vi "{{Msg}}Wrapper.vi"(6 "Error":errorcluster, 7 "Layer":T10, 9 "Payload":T9, 10 "MsgAttribs":T6 {"AbsoluteTime" format="%<%x %.3X>T"}, 11 "Actor":T1) -> (1 "Payload":T9, 2 "MsgAttribs":T6 {"AbsoluteTime" format="%<%x %.3X>T"}, 3 "Actor":T1, 4 "Error":errorcluster, 5 "Layer":T10)   [LabVIEW 2020, in "_Template.lvlib" / "{{Msg}}.lvlib"]
uses:
  {{Msg}}.lvlib
  ActorMsg/ActorMsg.lvclass
  jettl/jettl/Actor/Actor.lvclass
  jettl/jettl/Origin.ctl
  jettl/jettl/jettl.lvlib
  jettl/jettl/Lifecycle.ctl
  jettl/jettl/Metadata/Metadata.lvclass
  jettl/jettl/MsgAttribs.ctl
  jettl/jettl/Msg/Msg.lvclass
  jettl/jettl/Msg.ctl
  jettl/jettl/PostSetup.ctl
  jettl/jettl/PreSetup.ctl
  jettl/jettl/MsgNames.ctl
  jettl/jettl/ActorAttribs.ctl
  jettl/jettl/ChildActors.ctl
  jettl/jettl/Actor.ctl
  Payload.ctl
  jettl/jettl/Layer.ctl
  jettl/jettl/MsgExecuteType.ctl
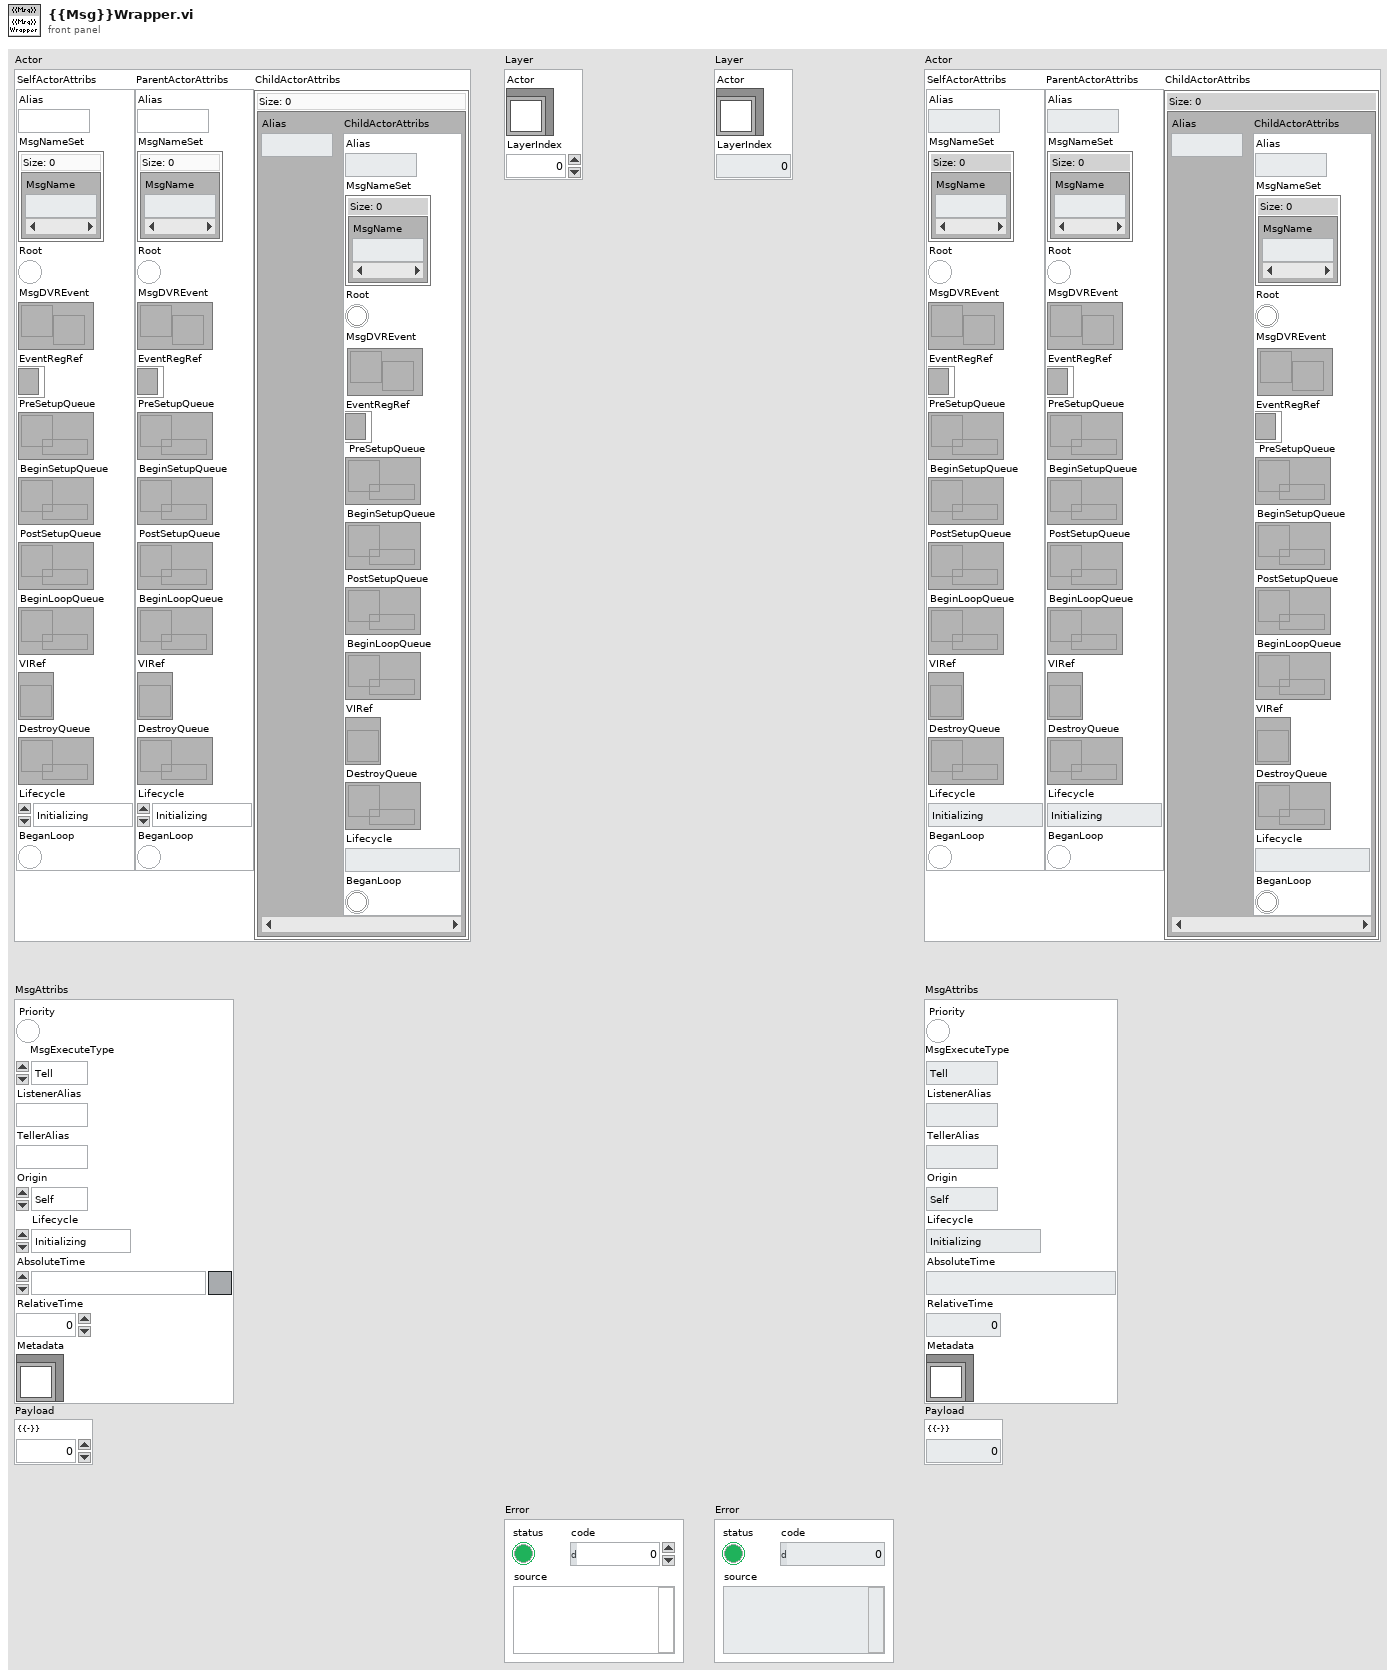
[diagram p1: front panel]
types:
  T1 = typedef "jettl.lvlib/Actor.ctl" = cluster{"SelfActorAttribs":T2, "ParentActorAttribs":T2, "ChildActorAttribs":T5}
  T2 = typedef "jettl.lvlib/ActorAttribs.ctl" = cluster{"Alias":string, "MsgNameSet":T3, "Root":bool, "MsgDVREvent":refnum<user-event>, "EventRegRef":refnum<event-registration>, "PreSetupQueue":refnum<queue>, "BeginSetupQueue":refnum<queue>, "PostSetupQueue":refnum<queue>, "BeginLoopQueue":refnum<queue>, "VIRef":refnum<vi>, "DestroyQueue":refnum<queue>, "Lifecycle":T4, "BeganLoop":bool}
  T3 = typedef "jettl.lvlib/MsgNames.ctl" = set{string}
  T4 = typedef "jettl.lvlib/Lifecycle.ctl" = enum16{"Initializing", "SettingUp", "Starting", "Running", "Stopping", "TearingDown", "Terminated"}
  T5 = typedef "jettl.lvlib/ChildActors.ctl" = map{string, T2}
  T6 = typedef "jettl.lvlib/MsgAttribs.ctl" = cluster{"Priority":bool, "MsgExecuteType":T7, "ListenerAlias":string, "TellerAlias":string, "Origin":T8, "Lifecycle":T4, "AbsoluteTime":timestamp, "RelativeTime":dbl, "Metadata":refnum<class "Metadata.lvclass">}
  T7 = typedef "jettl.lvlib/MsgExecuteType.ctl" = enum16{"Tell", "Call"}
  T8 = typedef "jettl.lvlib/Origin.ctl" = enum16{"Self", "Parent", "Child"}
  T9 = typedef "_Template.lvlib/{{Msg}}.lvlib/Payload.ctl" = cluster{"{{-}}":u8}
  T10 = typedef "jettl.lvlib/Layer.ctl" = cluster{"Actor":refnum<class "Actor.lvclass">, "LayerIndex":u8}
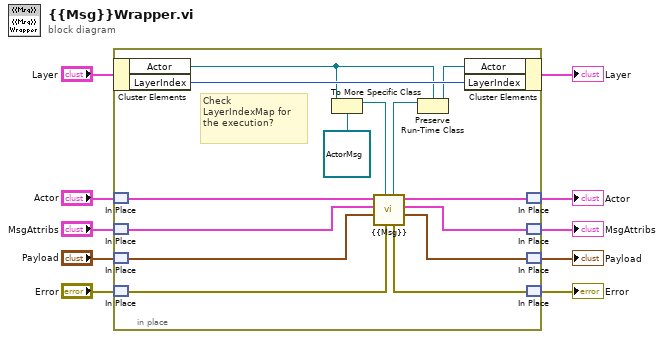
[diagram p0: block diagram]
diagram:
  n1 = in-place {
    # "Check LayerIndexMap for the execution?"
    n2 = in-place-cluster #1("Layer") -> ("Actor"=w14:refnum<class "Actor.lvclass">, "LayerIndex"=w24:u8)
    n3 = in-place-match #2("Actor") -> (w12:T1)
    n4 = in-place-match #3("MsgAttribs") -> (w18:T6)
    n5 = in-place-match #4("Payload") -> (w17:T9)
    n6 = in-place-match #5("Error") -> (w20:errorcluster)
    n7 = To More Specific Class(target class=refnum<class "ActorMsg.lvclass"> refnum ("_Template.lvlib:Templates.lvlib:TEMPLATE jettl Msg.lvlib:TEMPLATE jettl Msg.lvclass"), reference=w14) -> (specific class reference=w22:refnum<class "ActorMsg.lvclass">)  [unwired: 1 in, 1 out]
    n8 = call-dynamic "{{Msg}}.vi"("Error"=w20, "ActorMsg"=w22, "Payload"=w17, "MsgAttribs"=w18, "Actor"=w12) -> ("Payload"=w16:T9, "MsgAttribs"=w15:T6, "Actor"=w11:T1, "Error"=w19:errorcluster, "ActorMsg"=w21:refnum<class "ActorMsg.lvclass">)  [unwired: 2 in]
    n9 = Preserve Run-Time Class(object in=w21, 2:w14) -> (object out=w13:refnum<class "Actor.lvclass">)  [unwired: 1 in, 1 out]
    n10 = in-place-cluster #1("Actor"=w13, "LayerIndex"=w24) -> (→"Layer":T10)
    n11 = in-place-match #2(w11) -> (→"Actor":T1)
    n12 = in-place-match #3(w15) -> (→"MsgAttribs":T6)
    n13 = in-place-match #4(w16) -> (→"Payload":T9)
    n14 = in-place-match #5(w19) -> (→"Error":errorcluster)
  }
